vi "CVTEng UI.vi"() -> ()   [LabVIEW 2013, in "CVT Engine Editor.lvclass"]
doc: "UI that will be called when the node is selected."
uses:
  CVT Engine Editor.lvclass
  <vilib>/NI/Configuration Framework/Node/NodeRef.ctl
  <vilib>/NI/Configuration Framework/Node/NISE_CEF_Node.lvclass
  <vilib>/NI/AMC/Message Queue.ctl
  <vilib>/NI/AMC/Message.ctl
  <vilib>/NI/Tools/Keyed Array/KeyedArray.ctl
  <vilib>/NI/Configuration Framework/Node/UserEventRef.ctl
  <vilib>/NI/Configuration Framework/Controls/EventCluster.ctl
  <vilib>/NI/Configuration Framework/Node/RefreshUIEvent.ctl
  <vilib>/NI/Configuration Framework/Node/CacheState.ctl
  <vilib>/NI/Configuration Framework/Node/StopEvent.ctl
  <vilib>/NI/Configuration Framework/Node/NodeChangeEvent.ctl
  <vilib>/NI/Tag Bus Data Framework/Configuration Editor/Classes/Engine Parent/Engine Parent Editor Node.lvclass
  <vilib>/NI/Configuration Framework/serializable configuration/set alias.vi
  <vilib>/NI/Tools/Keyed Array/Tools_KeyedArray.lvlib
  <vilib>/NI/AMC/AMC.lvlib
  <vilib>/NI/Configuration Framework/NISE_CEF_TreeControl.lvlib
panel:
  in  "node change":T1
  in  "stop event":T2
  in  "cache state":T3
  in  "refresh UI":T4
  in  "user event":T5
  in  "main queue":T6
  in  "Name":string
  in  "node ref":T7
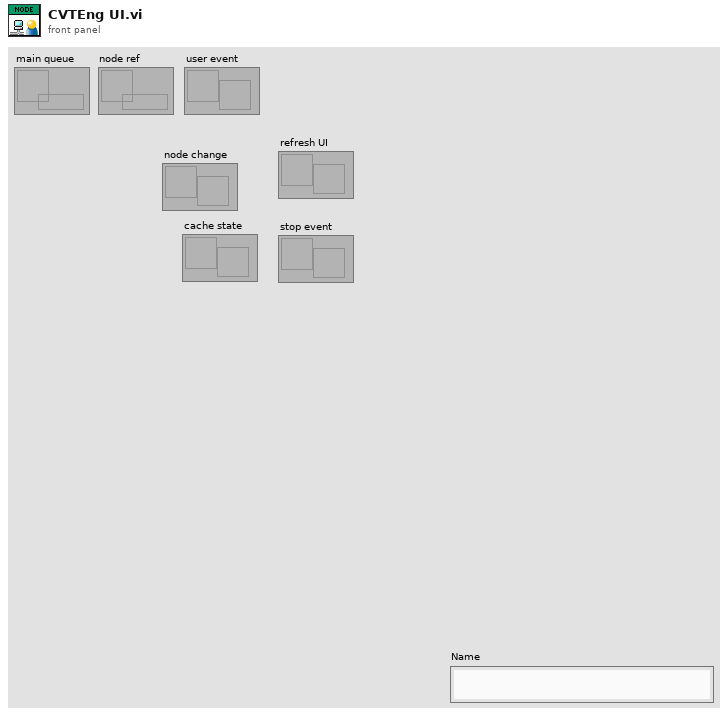
[diagram p1: front panel]
types:
  T1 = typedef "NISE_CEF_Node.lvclass/NodeChangeEvent.ctl" = refnum<user-event>
  T2 = typedef "NISE_CEF_Node.lvclass/StopEvent.ctl" = refnum<user-event>
  T3 = typedef "NISE_CEF_Node.lvclass/CacheState.ctl" = refnum<user-event>
  T4 = typedef "NISE_CEF_Node.lvclass/RefreshUIEvent.ctl" = refnum<user-event>
  T5 = typedef "NISE_CEF_Node.lvclass/UserEventRef.ctl" = refnum<user-event>
  T6 = typedef "AMC.lvlib/Message Queue.ctl" = refnum<queue>
  T7 = typedef "NISE_CEF_Node.lvclass/NodeRef.ctl" = refnum<data-value>
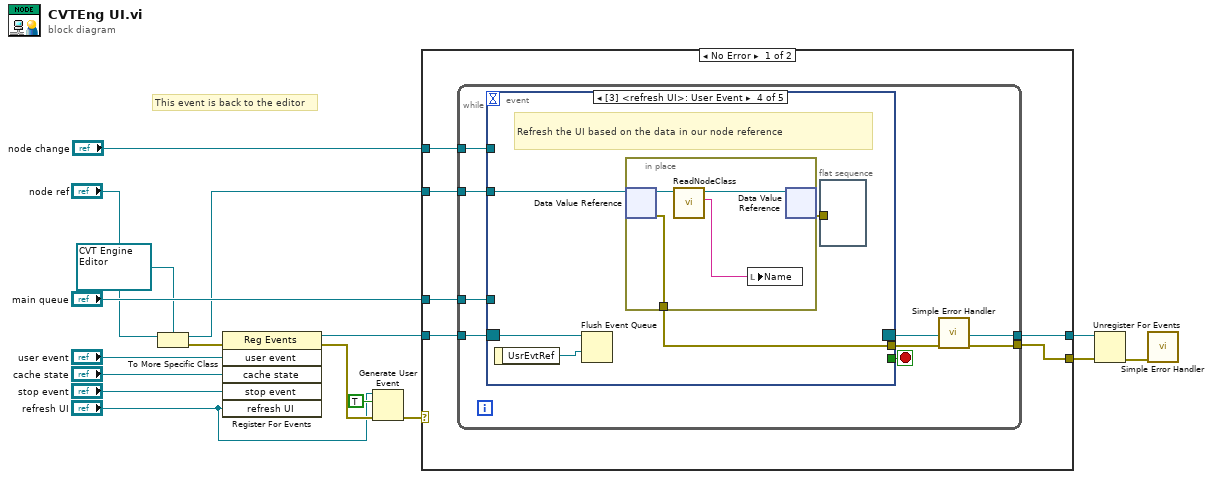
[diagram p0: block diagram]
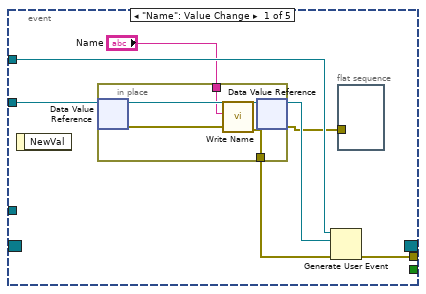
[diagram p2: hidden frame]
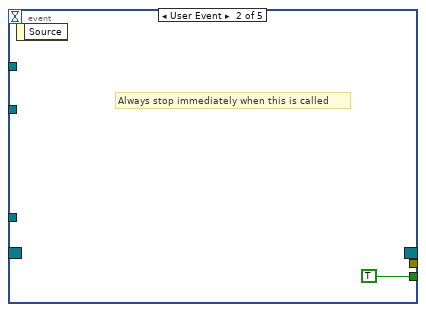
[diagram p3: hidden frame]
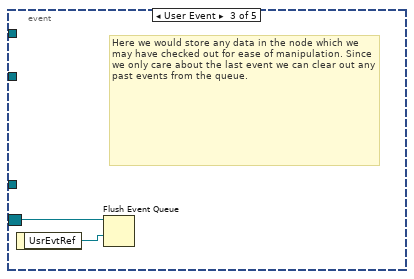
[diagram p4: hidden frame]
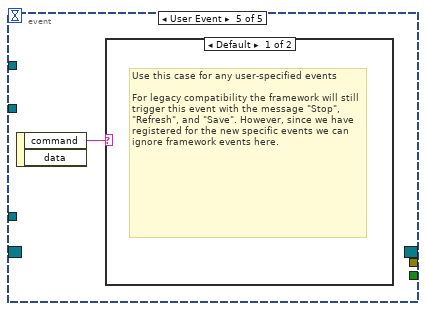
[diagram p5: hidden frame]
diagram:
  # "This event is back to the editor"
  n1 = To More Specific Class(target class=refnum<data-value> refnum, reference="node ref") -> (specific class reference=w1:refnum<data-value>, error out=w4:errorcluster)  [unwired: 1 in]
  n2 = register-events(error in=w4, "user event", "cache state", "stop event", "refresh UI") -> (reference out=w16:refnum<event-registration>, error out=w13:errorcluster)  [unwired: 1 in]
  n3 = Generate User Event(user event="refresh UI", event data cluster=TRUE ("event data"), error in=w13) -> (error out=w11:errorcluster)  [unwired: 1 in, 1 out]
  n4 = case shown="No Error" w11 {
    selector: w11 -> [_ w58]
    tunnel: w1 -> [w23 _]
    tunnel: "main queue" -> [w22 _]
    tunnel: w16 -> [w21 w57]
    tunnel: [w20 w57] -> w15
    tunnel: [w19 w58] -> w14
    tunnel: "node change" -> [w18 _]
    frame No Error {
      n5 = while {
        tunnel: w23 -> [w31]
        tunnel: w22 -> [w30]
        tunnel: w21 -> [w29]
        tunnel: [w28] -> w20
        tunnel: [w24] -> w19
        tunnel: w18 -> [w25]
        stop <- w26 stop-if-true
        n6 = event shown="[3] <refresh UI>: User Event" {
          selector: w29 -> [_ _ w46 w51 _]
          dyn-events: [_ _ _ _ _] -> w28
          timeout: _ -> [_ _ _ _ _]
          tunnel: w31 -> [w36 _ _ w47 _]
          tunnel: w30 -> [_ _ _ _ _]
          tunnel: [w38 _ _ w48 _] -> w27
          tunnel: [_ TRUE _ _ _] -> w26
          tunnel: w25 -> [w37 _ _ _ _]
          event "Name": Value Change {
            n7 = event-data() -> ()  [unwired: 1 in, 1 out]
            n8 = in-place {
              in-place-border: "Name" -> [w40]
              in-place-border: [w39] -> w32
              n9 = in-place-dvr #1(w36) -> (w43:refnum<class "CVT Engine Editor.lvclass">, w42:errorcluster)
              n10 = call <vilib>:"Write Name.vi"("error in"=w42, "Name"=w40, "Engine in"=w43) -> ("error out"=w39:errorcluster, "Engine out"=w41:refnum<class "CVT Engine Editor.lvclass">)  [unwired: 7 in]
              n11 = in-place-dvr #1(w41) -> (w35:refnum<data-value>, w33:errorcluster)
            }
            n12 = Generate User Event(user event=w37, event data cluster=w35, error in=w32) -> (error out=w38:errorcluster)  [unwired: 1 in, 1 out]
            n13 = flat-sequence {
              tunnel: w33 -> [_]
              frame #0 {
              }
            }
          }
          event User Event {
            # "Always stop immediately when this is called"
            n14 = event-data() -> ()  [unwired: 1 in, 1 out]
          }
          event User Event {
            # "Here we would store any data in the node which we may have checked out for ease of manipulation. Since we only care about the last event we can clear out any past events from the queue."
            n15 = event-data() -> ("UsrEvtRef"=w45:refnum<user-event>)  [unwired: 1 in]
            n16 = Flush Event Queue(0:w46, 2:w45) -> ()  [unwired: 4 in, 3 out]
          }
          event User Event {
            # "Refresh the UI based on the data in our node reference"
            n17 = event-data() -> ("UsrEvtRef"=w50:refnum<user-event>)  [unwired: 1 in]
            n18 = Flush Event Queue(0:w51, 2:w50) -> ()  [unwired: 4 in, 3 out]
            n19 = in-place {
              in-place-border: [w52] -> w48
              n20 = in-place-dvr #2(w47) -> (w55:refnum<class "CVT Engine Editor.lvclass">, w52:errorcluster)
              n21 = call <vilib>:"ReadNodeClass.vi"("node in"=w55) -> ("nodeClass"=w53:string, "node out"=w54:refnum<class "CVT Engine Editor.lvclass">)  [unwired: 8 in, 1 out]
              n22 = local write "Name"(w53) -> ()
              n23 = in-place-dvr #2(w54) -> (w49:errorcluster)  [unwired: 1 out]
            }
            n24 = flat-sequence {
              tunnel: w49 -> [_]
              frame #0 {
              }
            }
          }
          event User Event {
            n25 = event-data() -> ("command"=w56:string)  [unwired: 1 in, 1 out]
            n26 = case shown="Default" w56 {
              frame Default {
                # "Use this case for any user-specified events\n\nFor legacy compatibility the framework will still trigger this event with the message \"Stop\", \"Refresh\", and \"Save\". However, since we have registered for the new specific events we can ignore framework events here."
              }
              frame "Refresh", "Save", "Stop" {
              }
            }
          }
        }
        n27 = call <vilib>:"Simple Error Handler.vi"("error in (no error)"=w27) -> ("error out"=w24:errorcluster)  [unwired: 4 in, 4 out]
      }
    }
    frame Error {
    }
  }
  n28 = Unregister For Events(event registration refnum=w15, error in=w14) -> (error out=w10:errorcluster)
  n29 = call <vilib>:"Simple Error Handler.vi"("error in (no error)"=w10) -> ()  [unwired: 4 in, 5 out]
